vi "ALL VFunction.vi"(0 "VISA resource name":refnum<visa-resource-name>="DSOS404", 1 "txt path":string="D:\\TekScope\\DSOS404", 3 "TimeStampInput":string="201711091600DSOS404", 5 "error in (no error)":errorcluster) -> (14 "VISA resource name out":refnum<visa-resource-name>="DSOS404", 15 "Waveform Graph":waveform(dbl)[](graph)=[{"t0"=timestamp(-4.999682067241551e-07 s since 1904-01-01), "dt"=5e-11, "Y"=array[20000 elements]}, {"t0"=timestamp(0 s since 1904-01-01), "dt"=1.0, "Y"=[]}, {"t0"=timestamp(0 s since 1904-01-01), "dt"=1.0, "Y"=[]}, {"t0"=timestamp(0 s since 1904-01-01), "dt"=1.0, "Y"=[]}], 17 "Channel Index":cluster{bool, bool, bool, bool}={TRUE, FALSE, FALSE, FALSE}, 18 "Array 3":T1(array[cluster])=[{{"Channel 1"=9.99999e+37, "Channel 2"=0.0, "Channel 3"=0.0, "Channel 4"=0.0}}, {{"Channel 1"=2.15325e-08, "Channel 2"=0.0, "Channel 3"=0.0, "Channel 4"=0.0}}, {{"Channel 1"=0.0471, "Channel 2"=0.0, "Channel 3"=0.0, "Channel 4"=0.0}}, {{"Channel 1"=2.155708e-08, "Channel 2"=0.0, "Channel 3"=0.0, "Channel 4"=0.0}}, {{"Channel 1"=5.35312e-09, "Channel 2"=0.0, "Channel 3"=0.0, "Channel 4"=0.0}}], 19 "error out":errorcluster)   [LabVIEW 2018]
panel:
  # "CH1"
  # "CH2"
  # "CH3"
  # "CH4"
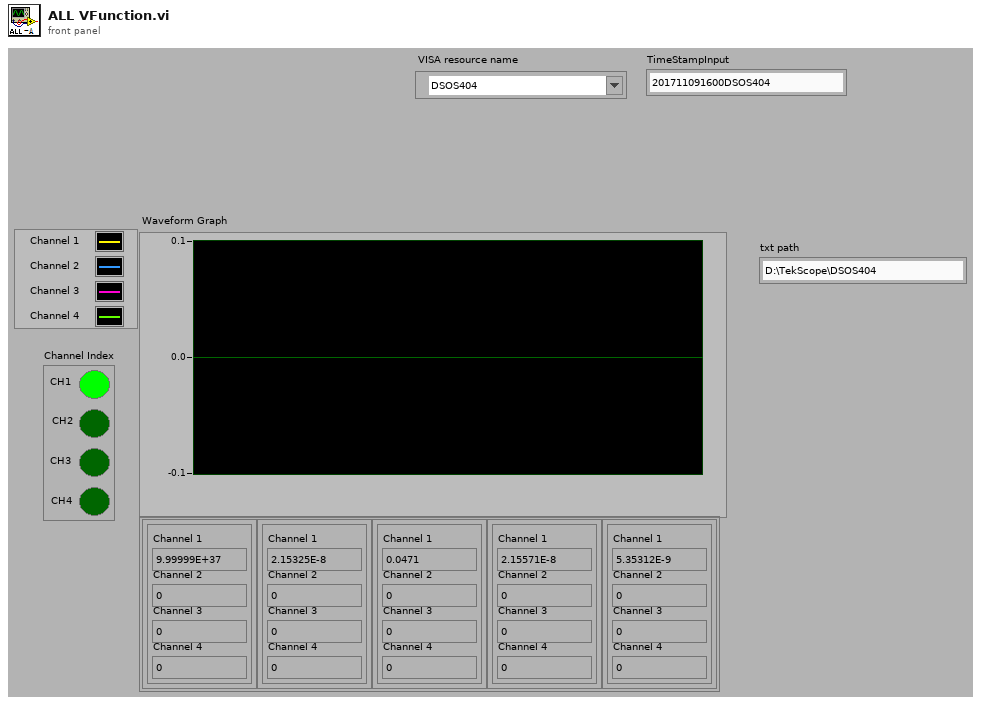
[diagram p1: front panel]
types:
  T1 = cluster{cluster{"Channel 1":dbl, "Channel 2":dbl, "Channel 3":dbl, "Channel 4":dbl}}[]
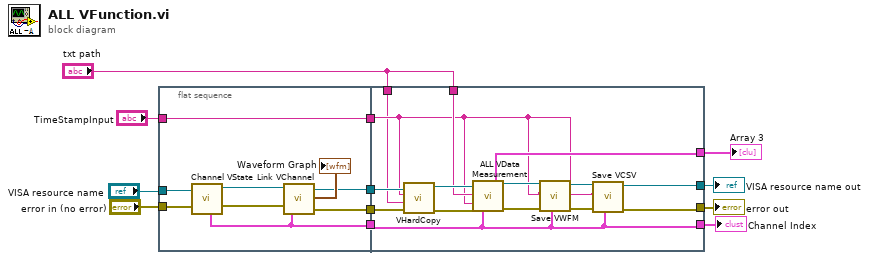
[diagram p0: block diagram]
diagram:
  n1 = flat-sequence {
    tunnel: [w19] -> w12
    tunnel: [w18] -> w11
    tunnel: "TimeStampInput" -> [w21]
    tunnel: "VISA resource name" -> [w17]
    tunnel: "error in (no error)" -> [w16]
    tunnel: [w21] -> w5
    tunnel: [w13] -> w4
    tunnel: [w24] -> w6
    tunnel: [w25] -> w7
    tunnel: w5 -> [w26]
    tunnel: w11 -> [w35]
    tunnel: w12 -> [w36]
    tunnel: w4 -> [w23]
    tunnel: [w23] -> w3
    tunnel: [w34] -> w2
    tunnel: "txt path" -> [w31]
    tunnel: "txt path" -> [w22]
    frame #0 {
      n2 = call "Channel VState.vi"("error in (no error)"=w16, "VISA resource name"=w17) -> ("error out"=w14:errorcluster, "Channel Index"=w13:cluster{bool, bool, bool, bool}, "VISA resource name 2"=w15:refnum<visa-resource-name>)  [unwired: 7 in]
      n3 = call "Link VChannel.vi"("Channel State"=w13, "error in (no error)"=w14, "VISA resource name"=w15) -> ("error out"=w18:errorcluster, "Waveform Graph"=→"Waveform Graph":waveform(dbl)[], "VISA resource name out"=w19:refnum<visa-resource-name>)  [unwired: 2 in]
    }
    frame #1 {
      n4 = call "VHardCopy.vi"("error in (no error)"=w35, "File path"=w22, "TimeStamp"=w26, "VISA resource name"=w36) -> ("error out"=w33:errorcluster, "VISA resource name out"=w32:refnum<visa-resource-name>)  [unwired: 6 in]
      n5 = call "ALL VData Measurement.vi"("VISA resource name"=w32, "txt path"=w31, "TimeStamp"=w26, "error in"=w33, "Channel State"=w23) -> ("VISA resource name out"=w30:refnum<visa-resource-name>, "Array"=w34:T1, "error out"=w29:errorcluster)  [unwired: 8 in]
      n6 = call "Save VWFM.vi"("Channel State"=w23, "error in (no error)"=w29, "TimeStamp"=w26, "VISA resource name"=w30) -> ("error out"=w27:errorcluster, "VISA resource name out"=w28:refnum<visa-resource-name>)  [unwired: 6 in]
      n7 = call "Save VCSV.vi"("Channel State"=w23, "error in (no error)"=w27, "TimeStamp"=w26, "VISA resource name"=w28) -> ("error out"=w24:errorcluster, "VISA resource name out"=w25:refnum<visa-resource-name>)  [unwired: 6 in]
    }
  }
  "VISA resource name out" <- w7
  "error out" <- w6
  "Channel Index" <- w3
  "Array 3" <- w2
